vi "New (8B).vi"(8 "error in (no error)":errorcluster, 10 "count (1)":u64=1, 11 "Pointer type":refnum<class "Pointer.lvclass">) -> (0 "error out":errorcluster, 3 "Pointer":refnum<class "Pointer.lvclass">)   [LabVIEW 2016, in "Memory Manager.lvlib" / "Pointer.lvclass"]
uses:
  Pointer.lvclass
  Pointer.lvclass/Pointer.ctl
  Set Address.vi
  Set Size.vi
  Set Internal.vi
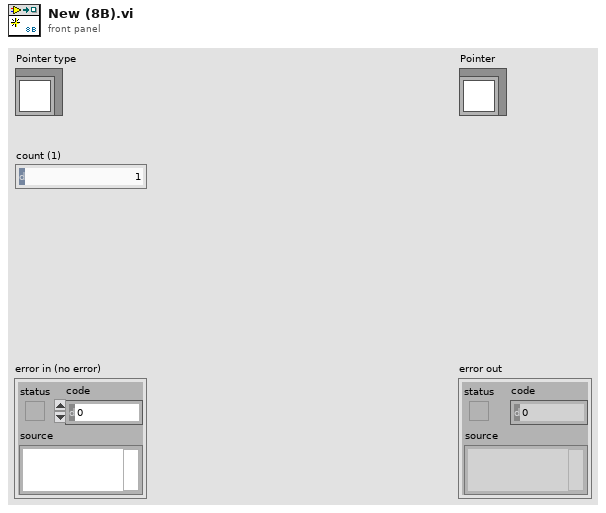
[diagram p1: front panel]
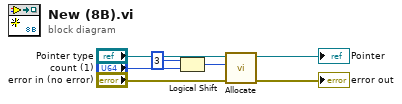
[diagram p0: block diagram]
diagram:
  n1 = Logical Shift(y=i16 3, x="count (1)") -> (x << y=w2:u64)
  n2 = call "Allocate.vi"("error in (no error)"="error in (no error)", "size"=w2, "Pointer in"="Pointer type") -> ("error out"=→"error out":errorcluster, "Pointer out"=→"Pointer":refnum<class "Pointer.lvclass">)  [unwired: 7 in]
